vi "Internecine Avoider.vi"(7 "net address":u32, 8 "error in (no error)":errorcluster, 11 "port":u16) -> (0 "error out":errorcluster, 3 "connection ID":refnum<k5>)   [LabVIEW 2011]
uses:
  TCP Listen List Operations.ctl
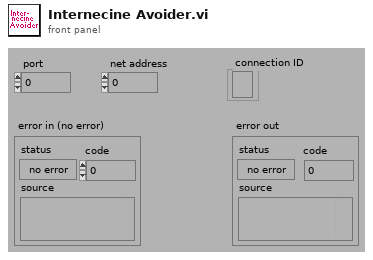
[diagram p1: front panel]
types:
  T1 = typedef "TCP Listen List Operations.ctl" = enum16{"Search", "Retrieve Element", "Add Element", "Delete Element"}
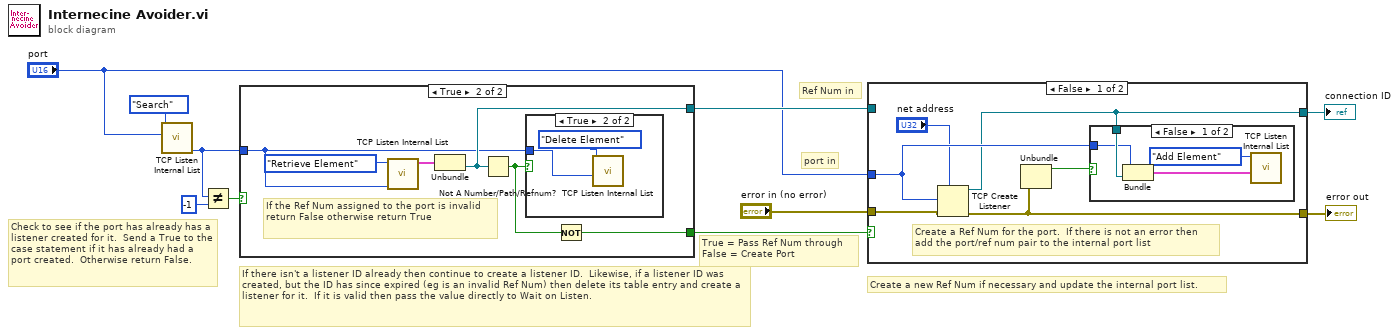
[diagram p0: block diagram]
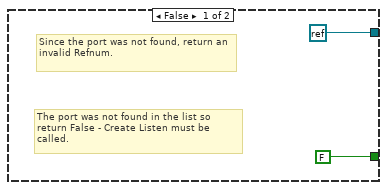
[diagram p4: hidden frame]
diagram:
  # "port in"
  # "Ref Num in"
  # "True = Pass Ref Num through\nFalse = Create Port"
  # "Create a new Ref Num if necessary and update the internal port list."
  # "If there isn't a listener ID already then continue to create a listener ID.  Likewise, if a listener ID was created, but the ID has since expired (eg is an invalid Ref Num) then delete its table entry and create a listener for it.  If it is valid then pass the value directly to Wait on Listen."
  # "Check to see if the port has already has a listener created for it.  Send a True to the case statement if it has already had a port created.  Otherwise return False."
  n1 = call "TCP Listen Internal List.vi"("Port"="port", "Operation"=TCP_Listen_List_Operations."Search") -> ("Element # \n(-1 if not found)"=w9:i32)  [unwired: 2 in, 7 out]
  n2 = Not Equal?(x=w9, y=-1) -> (x != y?=w4:bool)
  n3 = case shown="True" w4 {
    tunnel: w9 -> [_ w14]
    tunnel: [FALSE w16] -> w8
    tunnel: [refnum<k0> refnum w15] -> w7
    frame False {
      # "Since the port was not found, return an invalid Refnum."
      # "The port was not found in the list so return False - Create Listen must be called."
    }
    frame True {
      # "If the Ref Num assigned to the port is invalid return False otherwise return True"
      n4 = call "TCP Listen Internal List.vi"("Index #"=w14, "Operation"=TCP_Listen_List_Operations."Retrieve Element") -> ("Item Requested"=w18:cluster{u16, refnum<k5>})  [unwired: 2 in, 7 out]
      n5 = Unbundle(w18) -> (w15:refnum<k5>)  [unwired: 1 out]
      n6 = Not A Number/Path/Refnum?(number/path/refnum=w15) -> (NaN/Path/Refnum?=w17:bool)
      n7 = case shown="True" w17 {
        tunnel: w14 -> [_ w20]
        frame False {
        }
        frame True {
          n8 = call "TCP Listen Internal List.vi"("Index #"=w20, "Operation"=TCP_Listen_List_Operations."Delete Element") -> ()  [unwired: 2 in, 8 out]
        }
      }
      n9 = Not(x=w17) -> (.not. x?=w16:bool)
    }
  }
  n10 = case shown="False" w8 {
    tunnel: w7 -> [_ w32]
    tunnel: "port" -> [w24 _]
    tunnel: [w23 w32] -> w3
    tunnel: "error in (no error)" -> [w26 w31]
    tunnel: [w22 w31] -> w2
    frame False {
      # "Create a Ref Num for the port.  If there is not an error then\nadd the port/ref num pair to the internal port list"
      n11 = TCP Create Listener(7:"net address", 8:w26, 10:w24) -> (0:w22:errorcluster, 3:w23:refnum<k5>)  [unwired: 3 out]
      n12 = Unbundle(w22) -> ("status"=w25:bool)  [unwired: 2 out]
      n13 = case shown="False" w25 {
        tunnel: w24 -> [w29 _]
        tunnel: w23 -> [w30 _]
        frame False {
          n14 = Bundle("port"=w29, "listener ID"=w30) -> (w28:cluster{"port":u16, "listener ID":refnum<k5>})  [unwired: 1 out]
          n15 = call "TCP Listen Internal List.vi"("Element In"=w28, "Operation"=TCP_Listen_List_Operations."Add Element") -> ()  [unwired: 2 in, 8 out]
        }
        frame True {
        }
      }
    }
    frame True {
    }
  }
  "error out" <- w2
  "connection ID" <- w3
